vi "SMO.UI.TestLauncher.vi"() -> ()   [LabVIEW 2021, in "smo.lvlib" / "SMO.UI.lvclass"]
uses:
  SMO.UI.lvclass
  SMO.UI.lvclass/SMO.UI.ctl
  SMO/SMO.lvclass
  SMO/Typedefs/SMOState --Enum.ctl
  C:/Repositories/SMO/src/SMO/SMO.lvclass
  Typedefs/SMO.UI State--enum.ctl
panel:
  out "UI State":T1
  out "error out":errorcluster
  in  "Stop":bool
  # "SMO.UI Test Launcher"
  # "For instructions on how to use the JKI State Machine Objects, examples and video tutorials, visit:\nhttp://jki.net/state-machine-objects/\n\nJKI State Machine Objects™\nhttp://jki.net/state-machine-objects/\nCopyright (C) 2005-2015, JKI <info@jki.net>\nALL RIGHTS RESERVED"
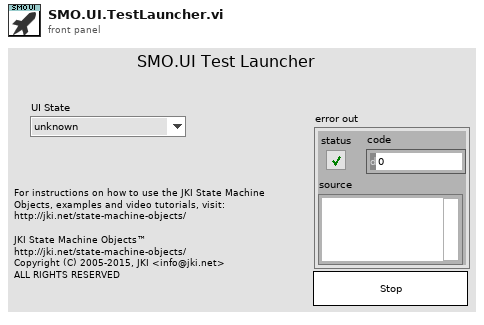
[diagram p1: front panel]
types:
  T1 = typedef "smo.lvlib/SMO.UI.lvclass/SMO.UI State--enum.ctl" = enum16{"unknown", "Opened", "Closed"}
  T2 = typedef "smo.lvlib/SMO.lvclass/Public Events.ctl" = cluster{"Error":refnum<user-event>, "State":refnum<user-event>, "Reserve State":refnum<user-event>}
  T3 = typedef "smo.lvlib/SMO.UI.lvclass/PublicEvents--Cluster.ctl" = cluster{"UI Hidden":refnum<user-event>, "UI State":refnum<user-event>}
  T4 = cluster{"Event Registration Refnum":refnum<event-registration>}
  T5 = typedef "smo.lvlib/SMO.lvclass/SMOState --Enum.ctl" = enum16{"unknown", "Created", "Started", "Stopped"}
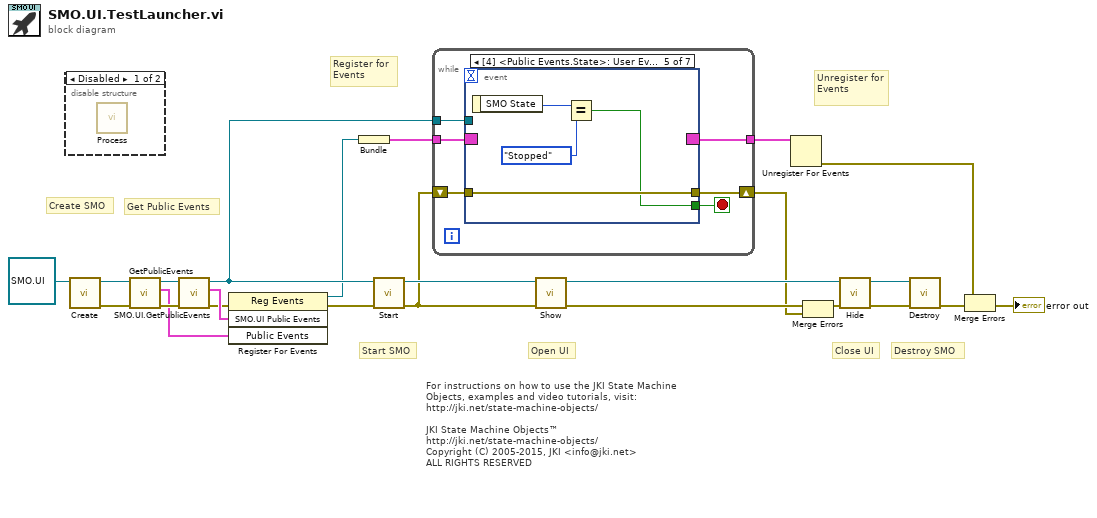
[diagram p0: block diagram]
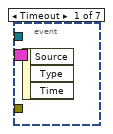
[diagram p3: hidden frame]
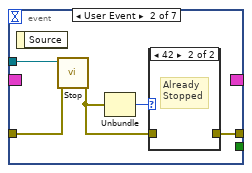
[diagram p4: hidden frame]
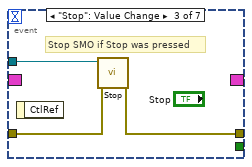
[diagram p6: hidden frame]
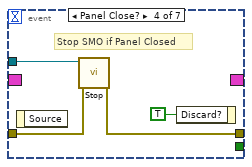
[diagram p7: hidden frame]
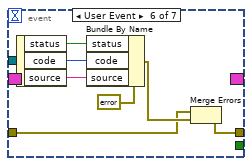
[diagram p8: hidden frame]
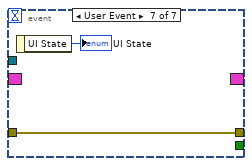
[diagram p9: hidden frame]
diagram:
  # "For instructions on how to use the JKI State Machine Objects, examples and video tutorials, visit:\nhttp://jki.net/state-machine-objects/\n\nJKI State Machine Objects™\nhttp://jki.net/state-machine-objects/\nCopyright (C) 2005-2015, JKI <info@jki.net>\nALL RIGHTS RESERVED"
  # "Get Public Events"
  # "Start SMO"
  # "Destroy SMO"
  # "Create SMO"
  # "Close UI"
  # "Open UI"
  # "Unregister for Events"
  # "Register for Events"
  n1 = disable-structure shown="Disabled" {
    frame Disabled {
      n2 = call-dynamic "Process.vi"() -> ()  [unwired: 10 in, 2 out]
    }
    frame Enabled {
    }
  }
  n3 = call "Create.vi"("SMO"=refnum<class "SMO.UI.lvclass"> refnum ("SMO.UI.lvclass")) -> ("error out"=w5:errorcluster, "SMO out"=w3:refnum<class "SMO.UI.lvclass">)  [unwired: 8 in, 1 out]
  n4 = call "GetPublicEvents.vi"("error in (no error)"=w5, "SMO"=w3) -> ("error out"=w4:errorcluster, "Public Events"=w1:T2, "SMO out"=w2:refnum<class "SMO.UI.lvclass">)  [unwired: 7 in]
  n5 = call "SMO.UI.GetPublicEvents.vi"("error in (no error)"=w4, "SMO.UI"=w2) -> ("error out"=w7:errorcluster, "SMO.UI Public Events"=w9:T3, "SMO.UI out"=w10:refnum<class "SMO.UI.lvclass">)  [unwired: 7 in]
  n6 = register-events(error in=w7, w9, w1) -> (reference out=w8:refnum<event-registration>, error out=w6:errorcluster)  [unwired: 1 in]
  n7 = Bundle("Event Registration Refnum"=w8) -> (w23:T4)  [unwired: 1 in]
  n8 = call "Start.vi"("error in (no error)"=w6, "SMO"=w10) -> ("error out"=w15:errorcluster, "SMO"=w22:refnum<class "SMO.UI.lvclass">)  [unwired: 8 in]
  n9 = while {
    shift-right: [w29] -> w14
    shift-left: w15 -> [w28]
    tunnel: w23 -> [w27]
    tunnel: [w26] -> w24
    tunnel: w10 -> [w25]
    stop <- w30 stop-if-true
    n10 = event shown="[4] <Public Events.State>: User Event" {
      selector: w27 -> [_ _ _ _ _ _ _]
      dyn-events: [_ _ _ _ _ _ _] -> w26
      timeout: _ -> [_ _ _ _ _ _ _]
      tunnel: [_ _ _ _ w44 _ _] -> w30
      tunnel: w25 -> [_ w35 w39 w43 _ _ _]
      tunnel: [_ w32 w38 w42 w45 w48 w56] -> w29
      tunnel: w28 -> [_ w34 w37 w41 w45 w49 w56]
      event Timeout {
        n11 = event-data() -> ()  [unwired: 1 in, 3 out]
      }
      event User Event {
        n12 = event-data() -> ()  [unwired: 1 in, 1 out]
        n13 = call "Stop.vi"("error in (no error)"=w34, "SMO"=w35) -> ("error out"=w31:errorcluster)  [unwired: 8 in, 1 out]
        n14 = Unbundle(w31) -> ("code"=w33:i32)  [unwired: 2 out]
        n15 = case shown="42" w33 {
          tunnel: w31 -> [w36 _]
          tunnel: [w36 _] -> w32
          frame Default {
          }
          frame 42 {
            # "Already\nStopped"
          }
        }
      }
      event "Stop": Value Change {
        # "Stop SMO if Stop was pressed"
        n16 = event-data() -> ()  [unwired: 1 in, 1 out]
        n17 = call "Stop.vi"("error in (no error)"=w37, "SMO"=w39) -> ("error out"=w38:errorcluster)  [unwired: 8 in, 1 out]
      }
      event Panel Close? {
        # "Stop SMO if Panel Closed"
        n18 = event-data() -> ()  [unwired: 1 in, 1 out]
        n19 = call "Stop.vi"("error in (no error)"=w41, "SMO"=w43) -> ("error out"=w42:errorcluster)  [unwired: 8 in, 1 out]
        n20 = event-data("Discard?"=TRUE ("OK")) -> ()  [unwired: 1 in, 1 out]
      }
      event User Event {
        n21 = event-data() -> ("SMO State"=w47:T5)  [unwired: 1 in]
        n22 = Equal?(x=w47, y=SMOState_--Enum."Stopped") -> (x = y?=w44:bool)
      }
      event User Event {
        n23 = event-data() -> ("status"=w54:bool, "code"=w53:i32, "source"=w52:string)  [unwired: 1 in]
        n24 = Bundle By Name(cluster=errorcluster {"status"=FALSE, "code"=0, "source"=""} ("error out"), "status"=w54, "code"=w53, "source"=w52) -> (w50:errorcluster)
        n25 = Merge Errors(w49, w50) -> (w48:errorcluster)
      }
      event User Event {
        n26 = event-data() -> ("UI State"=→"UI State":T1)  [unwired: 1 in]
      }
    }
  }
  n27 = call "Show.vi"("error in (no error)"=w15, "SMO.UI"=w22) -> ("error out"=w21:errorcluster, "SMO.UI out"=w20:refnum<class "SMO.UI.lvclass">)  [unwired: 8 in]
  n28 = Unregister For Events(event registration refnum=w24) -> (error out=w13:errorcluster)  [unwired: 1 in]
  n29 = Merge Errors(w21, w14) -> (w18:errorcluster)
  n30 = call "Hide.vi"("error in (no error)"=w18, "SMO.UI"=w20) -> ("error out"=w17:errorcluster, "SMO.UI out"=w19:refnum<class "SMO.UI.lvclass">)  [unwired: 8 in]
  n31 = call "Destroy.vi"("error in (no error)"=w17, "SMO"=w19) -> ("error out"=w11:errorcluster)  [unwired: 9 in]
  n32 = Merge Errors(w13, w11) -> (→"error out":errorcluster)
